vi "slider-check.vi"(0 "slider in":refnum<vi>, 1 "slider action":T1, 9 "slider from":refnum<vi>, 11 "value IN":dbl=5700.934579439253, 12 "default":dbl=5700.934579439253) -> (4 "slider out":refnum<vi>, 6 "max":dbl, 8 "rel OUT":dbl, 10 "min":dbl, 15 "value OUT":dbl=5700.934579439253)   [LabVIEW 2018]
uses:
  slider action.ctl
  Q - not nan -- real.vi
panel:
  in  "set step !":dbl(slide)=7372.0 min=0.0 max=16000.0 scale=0.0..16500.0
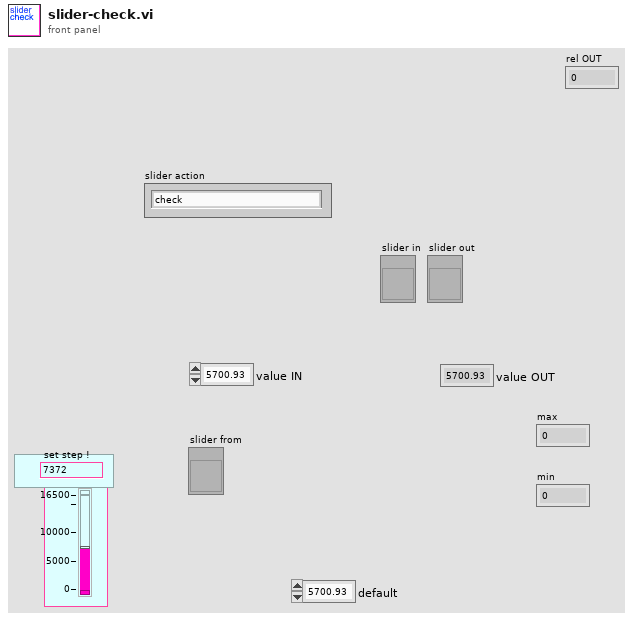
[diagram p1: front panel]
types:
  T1 = typedef "slider action.ctl" = enum16{"check", "copy range", "set from value", "set from ratio", "set from slider", "read using other slider"}
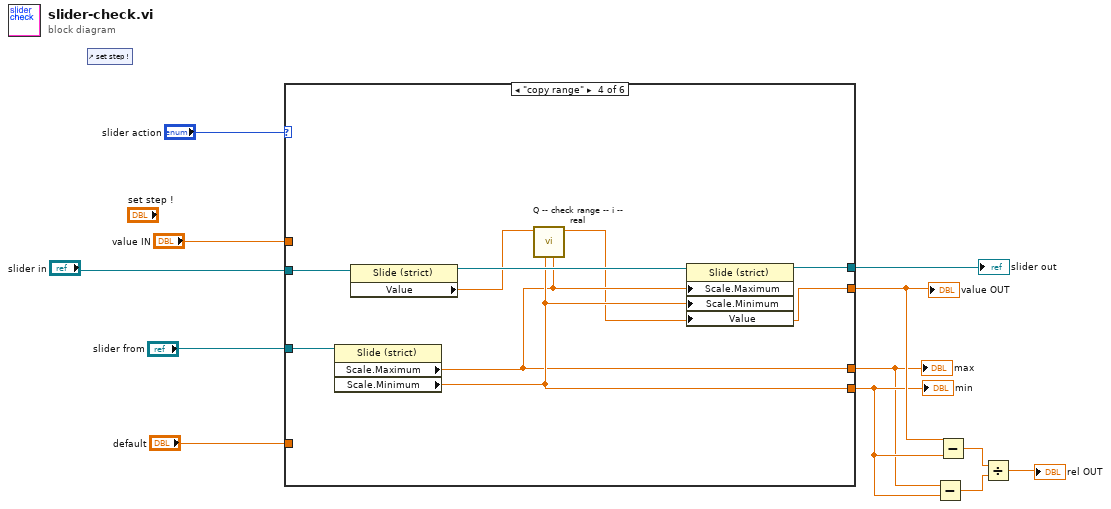
[diagram p0: block diagram]
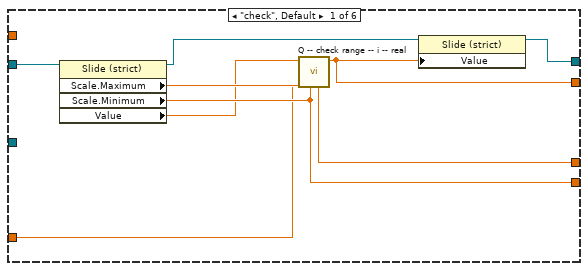
[diagram p2: hidden frame]
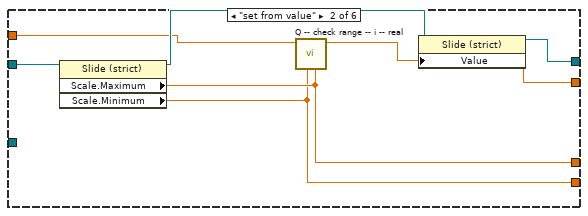
[diagram p3: hidden frame]
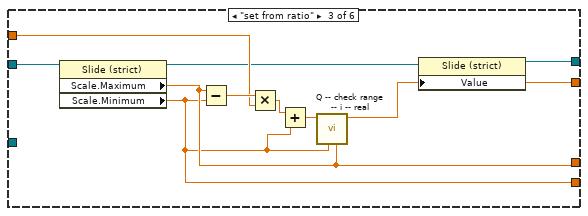
[diagram p4: hidden frame]
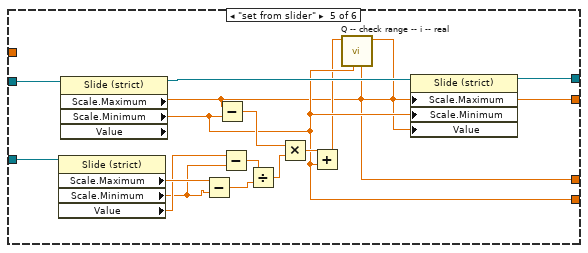
[diagram p5: hidden frame]
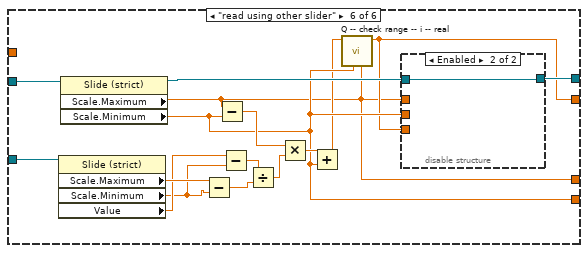
[diagram p6: hidden frame]
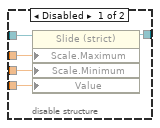
[diagram p7: hidden frame]
diagram:
  n1 = control-ref of="set step !"() -> ()  [unwired: 1 out]
  n2 = case shown="\"copy range\"" "slider action" {
    tunnel: "slider in" -> [w20 w27 w37 w43 w59 w75]
    tunnel: [w19 w26 w36 w38 w47 w63] -> w6
    tunnel: [w17 w24 w35 w44 w60 w76] -> w1
    tunnel: "slider from" -> [_ _ _ w45 w61 w77]
    tunnel: [w15 w22 w30 w40 w49 w65] -> w5
    tunnel: [w16 w23 w34 w39 w46 w62] -> w4
    tunnel: "value IN" -> [_ w21 w32 _ _ _]
    tunnel: "default" -> [w14 _ _ _ _ _]
    frame "check", Default {
      n3 = property class="Slide (strict)"(reference=w20) -> (reference out=w18:refnum<vi>, "Scale.Maximum"=w16:dbl, "Scale.Minimum"=w15:dbl, "Value"=w13:dbl)  [unwired: 1 in, 1 out]
      n4 = call "Q -- check range -- i -- real.vi"("upper"=w16, "lower"=w15, "default"=w14, "number"=w13) -> ("number in range"=w19:dbl)  [unwired: 5 in, 2 out]
      n5 = property class="Slide (strict)"(reference=w18, "Value"=w19) -> (reference out=w17:refnum<vi>)  [unwired: 1 in, 1 out]
    }
    frame "set from value" {
      n6 = property class="Slide (strict)"(reference=w27) -> (reference out=w25:refnum<vi>, "Scale.Maximum"=w23:dbl, "Scale.Minimum"=w22:dbl)  [unwired: 1 in, 1 out]
      n7 = call "Q -- check range -- i -- real.vi"("upper"=w23, "lower"=w22, "number"=w21) -> ("number in range"=w26:dbl)  [unwired: 6 in, 2 out]
      n8 = property class="Slide (strict)"(reference=w25, "Value"=w26) -> (reference out=w24:refnum<vi>)  [unwired: 1 in, 1 out]
    }
    frame "set from ratio" {
      n9 = property class="Slide (strict)"(reference=w37) -> (reference out=w31:refnum<vi>, "Scale.Maximum"=w34:dbl, "Scale.Minimum"=w30:dbl)  [unwired: 1 in, 1 out]
      n10 = Subtract(x=w34, y=w30) -> (x-y=w33:dbl)
      n11 = Multiply(x=w33, y=w32) -> (x*y=w29:dbl)
      n12 = Add(x=w29, y=w30) -> (x+y=w28:dbl)
      n13 = call "Q -- check range -- i -- real.vi"("upper"=w34, "lower"=w30, "number"=w28) -> ("number in range"=w36:dbl)  [unwired: 6 in, 2 out]
      n14 = property class="Slide (strict)"(reference=w31, "Value"=w36) -> (reference out=w35:refnum<vi>)  [unwired: 1 in, 1 out]
    }
    frame "copy range" {
      n15 = property class="Slide (strict)"(reference=w45) -> ("Scale.Maximum"=w39:dbl, "Scale.Minimum"=w40:dbl)  [unwired: 1 in, 2 out]
      n16 = property class="Slide (strict)"(reference=w43) -> (reference out=w42:refnum<vi>, "Value"=w41:dbl)  [unwired: 1 in, 1 out]
      n17 = call "Q -- check range -- i -- real.vi"("upper"=w39, "lower"=w40, "number"=w41) -> ("number in range"=w38:dbl)  [unwired: 6 in, 2 out]
      n18 = property class="Slide (strict)"(reference=w42, "Scale.Maximum"=w39, "Scale.Minimum"=w40, "Value"=w38) -> (reference out=w44:refnum<vi>)  [unwired: 1 in, 1 out]
    }
    frame "set from slider" {
      n19 = property class="Slide (strict)"(reference=w61) -> ("Scale.Maximum"=w57:dbl, "Scale.Minimum"=w55:dbl, "Value"=w56:dbl)  [unwired: 1 in, 2 out]
      n20 = property class="Slide (strict)" props=["Scale", "Maximum", "Scale", "Minimum", "Value"](reference=w59) -> (reference out=w58:refnum<vi>, "Scale.Maximum"=w46:dbl, "Scale.Minimum"=w49:dbl)  [unwired: 1 in, 2 out]
      n21 = Subtract(x=w57, y=w55) -> (x-y=w53:dbl)
      n22 = Subtract(x=w46, y=w49) -> (x-y=w51:dbl)
      n23 = Subtract(x=w56, y=w55) -> (x-y=w54:dbl)
      n24 = Divide(x=w54, y=w53) -> (x/y=w52:dbl)
      n25 = Multiply(x=w51, y=w52) -> (x*y=w50:dbl)
      n26 = Add(x=w50, y=w49) -> (x+y=w48:dbl)
      n27 = call "Q -- check range -- i -- real.vi"("upper"=w46, "lower"=w49, "number"=w48) -> ("number in range"=w47:dbl)  [unwired: 6 in, 2 out]
      n28 = property class="Slide (strict)"(reference=w58, "Scale.Maximum"=w46, "Scale.Minimum"=w49, "Value"=w47) -> (reference out=w60:refnum<vi>)  [unwired: 1 in, 1 out]
    }
    frame "read using other slider" {
      n29 = property class="Slide (strict)"(reference=w77) -> ("Scale.Maximum"=w73:dbl, "Scale.Minimum"=w71:dbl, "Value"=w72:dbl)  [unwired: 1 in, 2 out]
      n30 = property class="Slide (strict)"(reference=w75) -> (reference out=w74:refnum<vi>, "Scale.Maximum"=w62:dbl, "Scale.Minimum"=w65:dbl)  [unwired: 1 in, 1 out]
      n31 = Subtract(x=w73, y=w71) -> (x-y=w69:dbl)
      n32 = Subtract(x=w62, y=w65) -> (x-y=w67:dbl)
      n33 = Subtract(x=w72, y=w71) -> (x-y=w70:dbl)
      n34 = Divide(x=w70, y=w69) -> (x/y=w68:dbl)
      n35 = Multiply(x=w67, y=w68) -> (x*y=w66:dbl)
      n36 = Add(x=w66, y=w65) -> (x+y=w64:dbl)
      n37 = call "Q -- check range -- i -- real.vi"("upper"=w62, "lower"=w65, "number"=w64) -> ("number in range"=w63:dbl)  [unwired: 6 in, 2 out]
      n38 = disable-structure shown="Enabled" {
        disable-tunnel: [w82 w83] -> w76
        disable-tunnel: w74 -> [w81 w83]
        disable-tunnel: w65 -> [w80 _]
        disable-tunnel: w63 -> [w79 _]
        disable-tunnel: w62 -> [w78 _]
        frame Disabled {
          n39 = property class="Slide (strict)"(reference=w81, "Scale.Maximum"=w78, "Scale.Minimum"=w80, "Value"=w79) -> (reference out=w82:refnum<vi>)  [unwired: 1 in, 1 out]
        }
        frame Enabled {
        }
      }
    }
  }
  "value OUT" <- w6
  "min" <- w5
  "max" <- w4
  "slider out" <- w1
  n40 = Subtract(x=w4, y=w5) -> (x-y=w7:dbl)
  n41 = Subtract(x=w6, y=w5) -> (x-y=w8:dbl)
  n42 = Divide(x=w8, y=w7) -> (x/y=→"rel OUT":dbl)
